vi "Write_RoutineControl.vi"(8 "error in (no error)":errorcluster, 10 "RoutineControl":T1, 11 "AutoSubroutine in":refnum<class "AutoSubroutine.lvclass">) -> (0 "error out":errorcluster, 3 "AutoSubroutine out":refnum<class "AutoSubroutine.lvclass">)   [LabVIEW 2017, in "AutoSubroutine.lvclass"]
uses:
  AutoSubroutine.lvclass
  RoutineControl.ctl
  AutoSubroutine.lvclass/AutoSubroutine.ctl
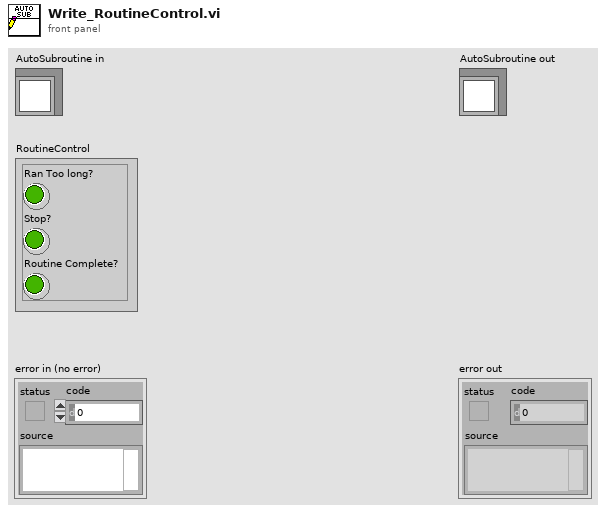
[diagram p1: front panel]
types:
  T1 = typedef "AutoSubroutine.lvclass/RoutineControl.ctl" = cluster{"Ran Too long?":bool, "Stop?":bool, "Routine Complete?":bool}
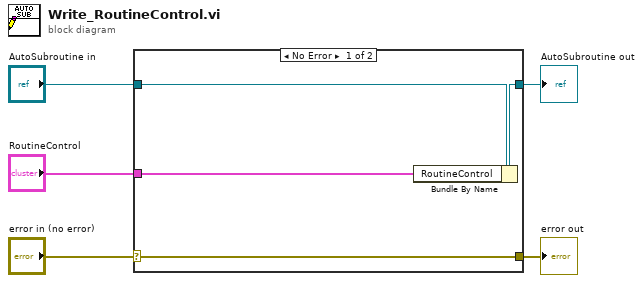
[diagram p0: block diagram]
diagram:
  n1 = case shown="No Error" "error in (no error)" {
    selector: "error in (no error)" -> [w9 w10]
    tunnel: [w9 w10] -> w4
    tunnel: [w7 w11] -> w2
    tunnel: "AutoSubroutine in" -> [w8 w11]
    tunnel: "RoutineControl" -> [w6 _]
    frame No Error {
      n2 = Bundle By Name(cluster=w8, "RoutineControl"=w6) -> (w7:refnum<class "AutoSubroutine.lvclass">)
    }
    frame Error {
    }
  }
  "error out" <- w4
  "AutoSubroutine out" <- w2
